vi "Set Data Ready Call Back.vi"(10 "datacallback":cluster{}, 11 "ppara":u32) -> (3 "ppara out":u32)   [LabVIEW 2021, in "vmmso.lvlib"]
doc: "DLL_API void WINAPI SetDataReadyCallBack(void* ppara, DataReadyCallBack datacallback);"
uses:
  vmmso.lvlib
  vmmso.dll
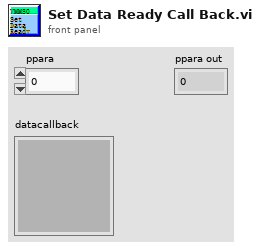
[diagram p1: front panel]
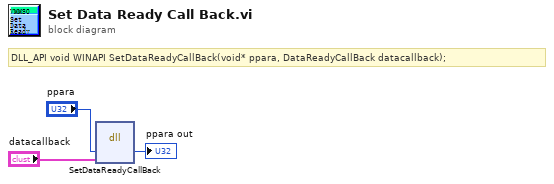
[diagram p0: block diagram]
diagram:
  # "DLL_API void WINAPI SetDataReadyCallBack(void* ppara, DataReadyCallBack datacallback);"
  n1 = dll-call lib="D:/labviewdemo/LabviewDemo 21/vmmso/vmmso.*" fn="SetDataReadyCallBack"("ppara"="ppara", "datacallback"="datacallback") -> ("ppara"=→"ppara out":u32)  [unwired: 5 in, 2 out]
